vi "AB_Log_Linker_Item_No_Class.vi"(6 "inclusion":T1, 7 "comment":string, 8 "error in (no error)":errorcluster, 9 "index":i32, 10 "linkerItem":T3) -> (0 "error out":errorcluster)   [LabVIEW 2020]
uses:
  <vilib>/Utility/lvfile.llb/LVFileType.ctl
  <vilib>/AppBuilder/Engine/AB_Engine_Linker_Inclusion.ctl
  <vilib>/Utility/lvfile.llb/NI_FileType.lvlib
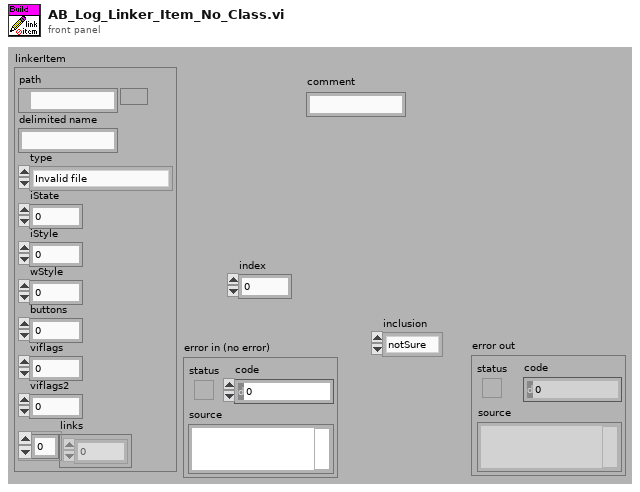
[diagram p1: front panel]
types:
  T1 = typedef "AB_Engine_Linker_Inclusion.ctl" = enum16{"notSure", "include", "exclude", "excludeChild"}
  T2 = typedef "NI_FileType.lvlib/LVFileType.ctl" = enum32{"Invalid file", "Unknown type", "Instrument", "Control", "Polymorphic VI", "Project", "Library", "LVClass", "XControl", "XNode", "Shared library", ".NET assembly", "ActiveX interface", "CIN", "Run-time menu", "Palette menu", "Help file", "LLB", "XNode Edit Dependency", "Class Private Data Control", "Statechart", "MathScript .m file", "Ladder Diagram", "LVLibp", "XNode Build Dependency"}
  T3 = cluster{"path":path, "delimited name":string, "type":T2, "iState":u32, "iStyle":u16, "wStyle":u16, "buttons":u16, "viflags":u32, "viflags2":u32, "links":u32[]}
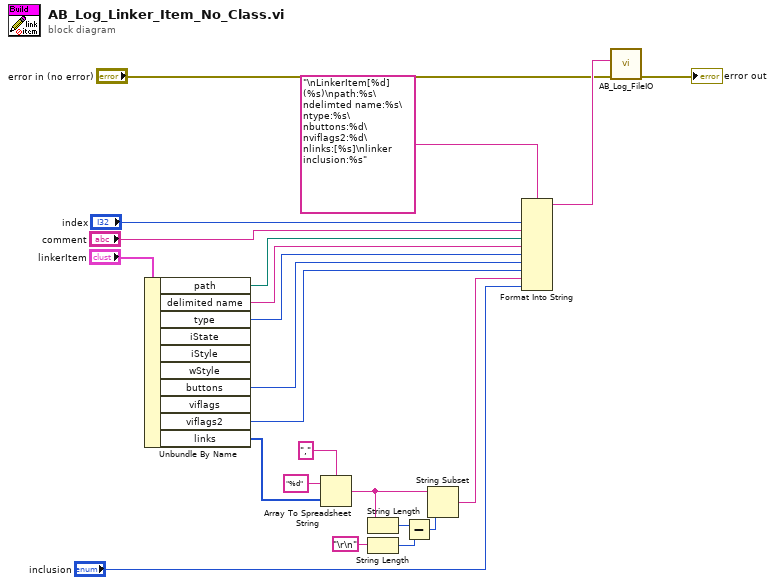
[diagram p0: block diagram]
diagram:
  n1 = Unbundle By Name("linkerItem") -> ("path"=w14:path, "delimited name"=w13:string, "type"=w12:T2, "buttons"=w11:u16, "viflags2"=w10:u32, "links"=w15:u32[])  [unwired: 4 out]
  n2 = Array To Spreadsheet String(delimiter (Tab)=",", array=w15, 3:"%d" ("format string")) -> (spreadsheet string=w2:string)
  n3 = String Length(string=w2) -> (length=w5:i32)
  n4 = String Length(string="\r\n") -> (length=w4:i32)
  n5 = Subtract(x=w5, y=w4) -> (x-y=w3:i32)
  n6 = String Subset(string=w2, length (rest)=w3) -> (substring=w1:string)  [unwired: 1 in]
  n7 = Format Into String(format string="\nLinkerItem[%d] (%s)\npath:%s\ndelimted name:%s\ntype:%s\nbuttons:%d\nviflags2:%d\nlinks:[%s]\nlinker inclusion:%s", "index", "comment", w14, w13, w12, w11, w10, w1, "inclusion") -> (resulting string=w21:string)  [unwired: 2 in, 1 out]
  n8 = call <vilib>:"AB_Log_FileIO.vi"("error in (no error)"="error in (no error)", "data"=w21) -> ("error out"=→"error out":errorcluster)  [unwired: 9 in]
